vi "S-N.vi"(10 "noise":waveform(dbl) caption="噪声输入", 11 "signal":waveform(dbl) caption="信号输入") -> (1 "信噪比(dB)":dbl, 2 "噪声平均功率":dbl, 3 "信号平均功率":dbl)   [LabVIEW 2018]
uses:
  <vilib>/measure/madcrms.llb/Basic Averaged DC-RMS for 1 Chan.vi
  <vilib>/measure/NI_MAPro.lvlib
panel:
  # "输入：信号波形与噪声波形\n输出：信噪比，信号和噪声平均功率"
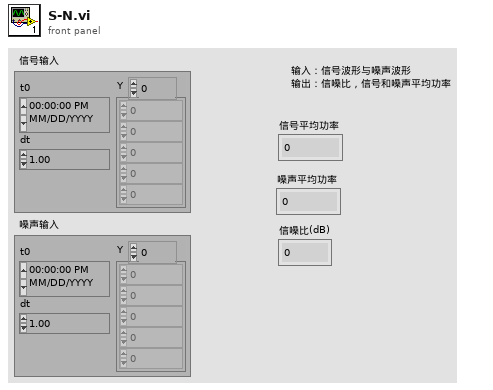
[diagram p1: front panel]
types:
  T1 = enum16{"Rectangular (none)", "Hanning", "Low side lobe"}
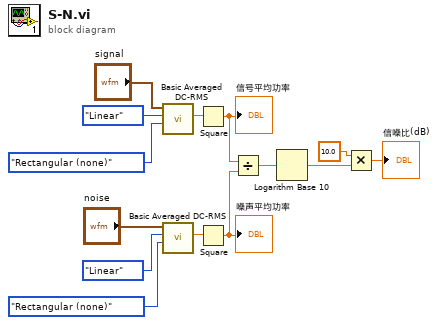
[diagram p0: block diagram]
diagram:
  n1 = call-poly <vilib>:"Basic Averaged DC-RMS.vi"("window"=T1."Rectangular (none)", "averaging type"=enum16{"Linear", "Exponential"}."Linear", "signal in"="signal") -> ("RMS value"=w9:dbl)  [unwired: 5 in, 3 out]
  n2 = call-poly <vilib>:"Basic Averaged DC-RMS.vi"("window"=T1."Rectangular (none)", "averaging type"=enum16{"Linear", "Exponential"}."Linear", "signal in"="noise") -> ("RMS value"=w14:dbl)  [unwired: 5 in, 3 out]
  n3 = Square(x=w9) -> (x^2=w6:dbl)
  "信号平均功率" <- w6
  n4 = Square(x=w14) -> (x^2=w5:dbl)
  "噪声平均功率" <- w5
  n5 = Divide(x=w6, y=w5) -> (x/y=w4:dbl)
  n6 = Logarithm Base 10(1:w4) -> (0:w3:dbl)
  n7 = Multiply(x=10.0, y=w3) -> (x*y=→"信噪比(dB)":dbl)
